vi "DeleteLayer.vi"(6 "error in":errorcluster, 7 "AntsRect":T8, 9 "Data in":T1={"Class"={"Ants"=refnum, "Layer"=refnum, "Templates"=refnum, "Icon"=refnum, "Glyph"=refnum, "Settings"=refnum, "Tools"=refnum, "History"=refnum}, "Ref"={"Add Layer"=refnum, "Remove Layer"=refnum, "Line Text"=[], "Body Text Spec"=refnum, "DNL_Font"=refnum, "glyph path str"=refnum, "templates path str"=refnum, "Arrow Up"=refnum, "Arrow Down"=refnum, "IE VI Ref"=refnum, "Glyphs tree"=refnum, "Templates tree"=refnum, "Layer Icon Text"=refnum, "Layer Template"=refnum, "Body Text"=refnum, "Search Templates"=refnum, "TextMarker"=refnum, "Tab Control"=refnum, "Search Glyphs"=refnum, "Line Color"=refnum, "DNL_Glyphs []"=refnum, "Fill Color"=refnum, "Tools"=refnum, "Icon"=refnum, "Preview"=refnum, "Ants"=refnum, "Terminals"=refnum, "menu reference"=refnum, "LayerNames"=[], "GlyphLoadAnimation"=refnum, "TemplateLoadAnimation"=refnum, "refreshGlyphs"=refnum, "refreshTemplates"=refnum}, "Support"={"AntsRect"={"left"=0, "top"=0, "right"=0, "bottom"=0}, "Mouse Move Coords"={"Horizontal"=0, "Vertical"=0}, "Mouse Down Coords"={"Horizontal"=0, "Vertical"=0}, "Temp Coord"={"Horizontal"=0, "Vertical"=0}, "Action"=enum."Default", "Edge Color"=4914962, "Fill Color"=16860, "Mouse Down?"=FALSE, "Draft Mode?"=FALSE, "Temp Icon"=bytes[3102], "CTRL Pressed"=FALSE, "Move Selection?"=FALSE, "AntsRect Orig"={"left"=0, "top"=0, "right"=0, "bottom"=0}, "Text"="", "TM Set?"=FALSE, "Mouse inside icon?"=FALSE, "Tool (old value)"=0, "Pencil Move Color"=0, "Swap Colors?"=FALSE, "Shift pressed?"=FALSE}}) -> (0 "error out":errorcluster, 3 "Data out":T1={"Class"={"Ants"=refnum, "Layer"=refnum, "Templates"=refnum, "Icon"=refnum, "Glyph"=refnum, "Settings"=refnum, "Tools"=refnum, "History"=refnum}, "Ref"={"Add Layer"=refnum, "Remove Layer"=refnum, "Line Text"=[], "Body Text Spec"=refnum, "DNL_Font"=refnum, "glyph path str"=refnum, "templates path str"=refnum, "Arrow Up"=refnum, "Arrow Down"=refnum, "IE VI Ref"=refnum, "Glyphs tree"=refnum, "Templates tree"=refnum, "Layer Icon Text"=refnum, "Layer Template"=refnum, "Body Text"=refnum, "Search Templates"=refnum, "TextMarker"=refnum, "Tab Control"=refnum, "Search Glyphs"=refnum, "Line Color"=refnum, "DNL_Glyphs []"=refnum, "Fill Color"=refnum, "Tools"=refnum, "Icon"=refnum, "Preview"=refnum, "Ants"=refnum, "Terminals"=refnum, "menu reference"=refnum, "LayerNames"=[], "GlyphLoadAnimation"=refnum, "TemplateLoadAnimation"=refnum, "refreshGlyphs"=refnum, "refreshTemplates"=refnum}, "Support"={"AntsRect"={"left"=0, "top"=0, "right"=0, "bottom"=0}, "Mouse Move Coords"={"Horizontal"=0, "Vertical"=0}, "Mouse Down Coords"={"Horizontal"=0, "Vertical"=0}, "Temp Coord"={"Horizontal"=0, "Vertical"=0}, "Action"=enum."Default", "Edge Color"=4914962, "Fill Color"=16860, "Mouse Down?"=FALSE, "Draft Mode?"=FALSE, "Temp Icon"=bytes[3102], "CTRL Pressed"=FALSE, "Move Selection?"=FALSE, "AntsRect Orig"={"left"=0, "top"=0, "right"=0, "bottom"=0}, "Text"="", "TM Set?"=FALSE, "Mouse inside icon?"=FALSE, "Tool (old value)"=0, "Pencil Move Color"=0, "Swap Colors?"=FALSE, "Shift pressed?"=FALSE}})   [LabVIEW 2020]
uses:
  Class/Ants/Ants.lvclass
  Class/FakedArray/FakedArray.lvclass
  vi.lib/LabVIEW Icon API/lv_icon/Classes/Icon/Icon.lvclass
  Class/Icon Library/Glyph.lvclass
  Class/Settings/Settings.lvclass
  Class/Tools/Tools Paint.lvclass
  History/History/History.lvclass
  vi.lib/LabVIEW Icon API/lv_icon/Classes/Layer/Layer.lvclass
  vi.lib/LabVIEW Icon API/LabVIEW Icon API.lvlib
  lv_icon.lvlib
  History/History.lvlib
  <vilib>/Utility/miscctls.llb/LVPoint32TypeDef.ctl
  Controls/SupportClass_Action.ctl
  vi.lib/LabVIEW Icon API/lv_icon/Controls/IEColor.ctl
  Controls/Support Cluster.ctl
  Controls/References Cluster.ctl
  Controls/IE Classes.ctl
  Controls/Global Data.ctl
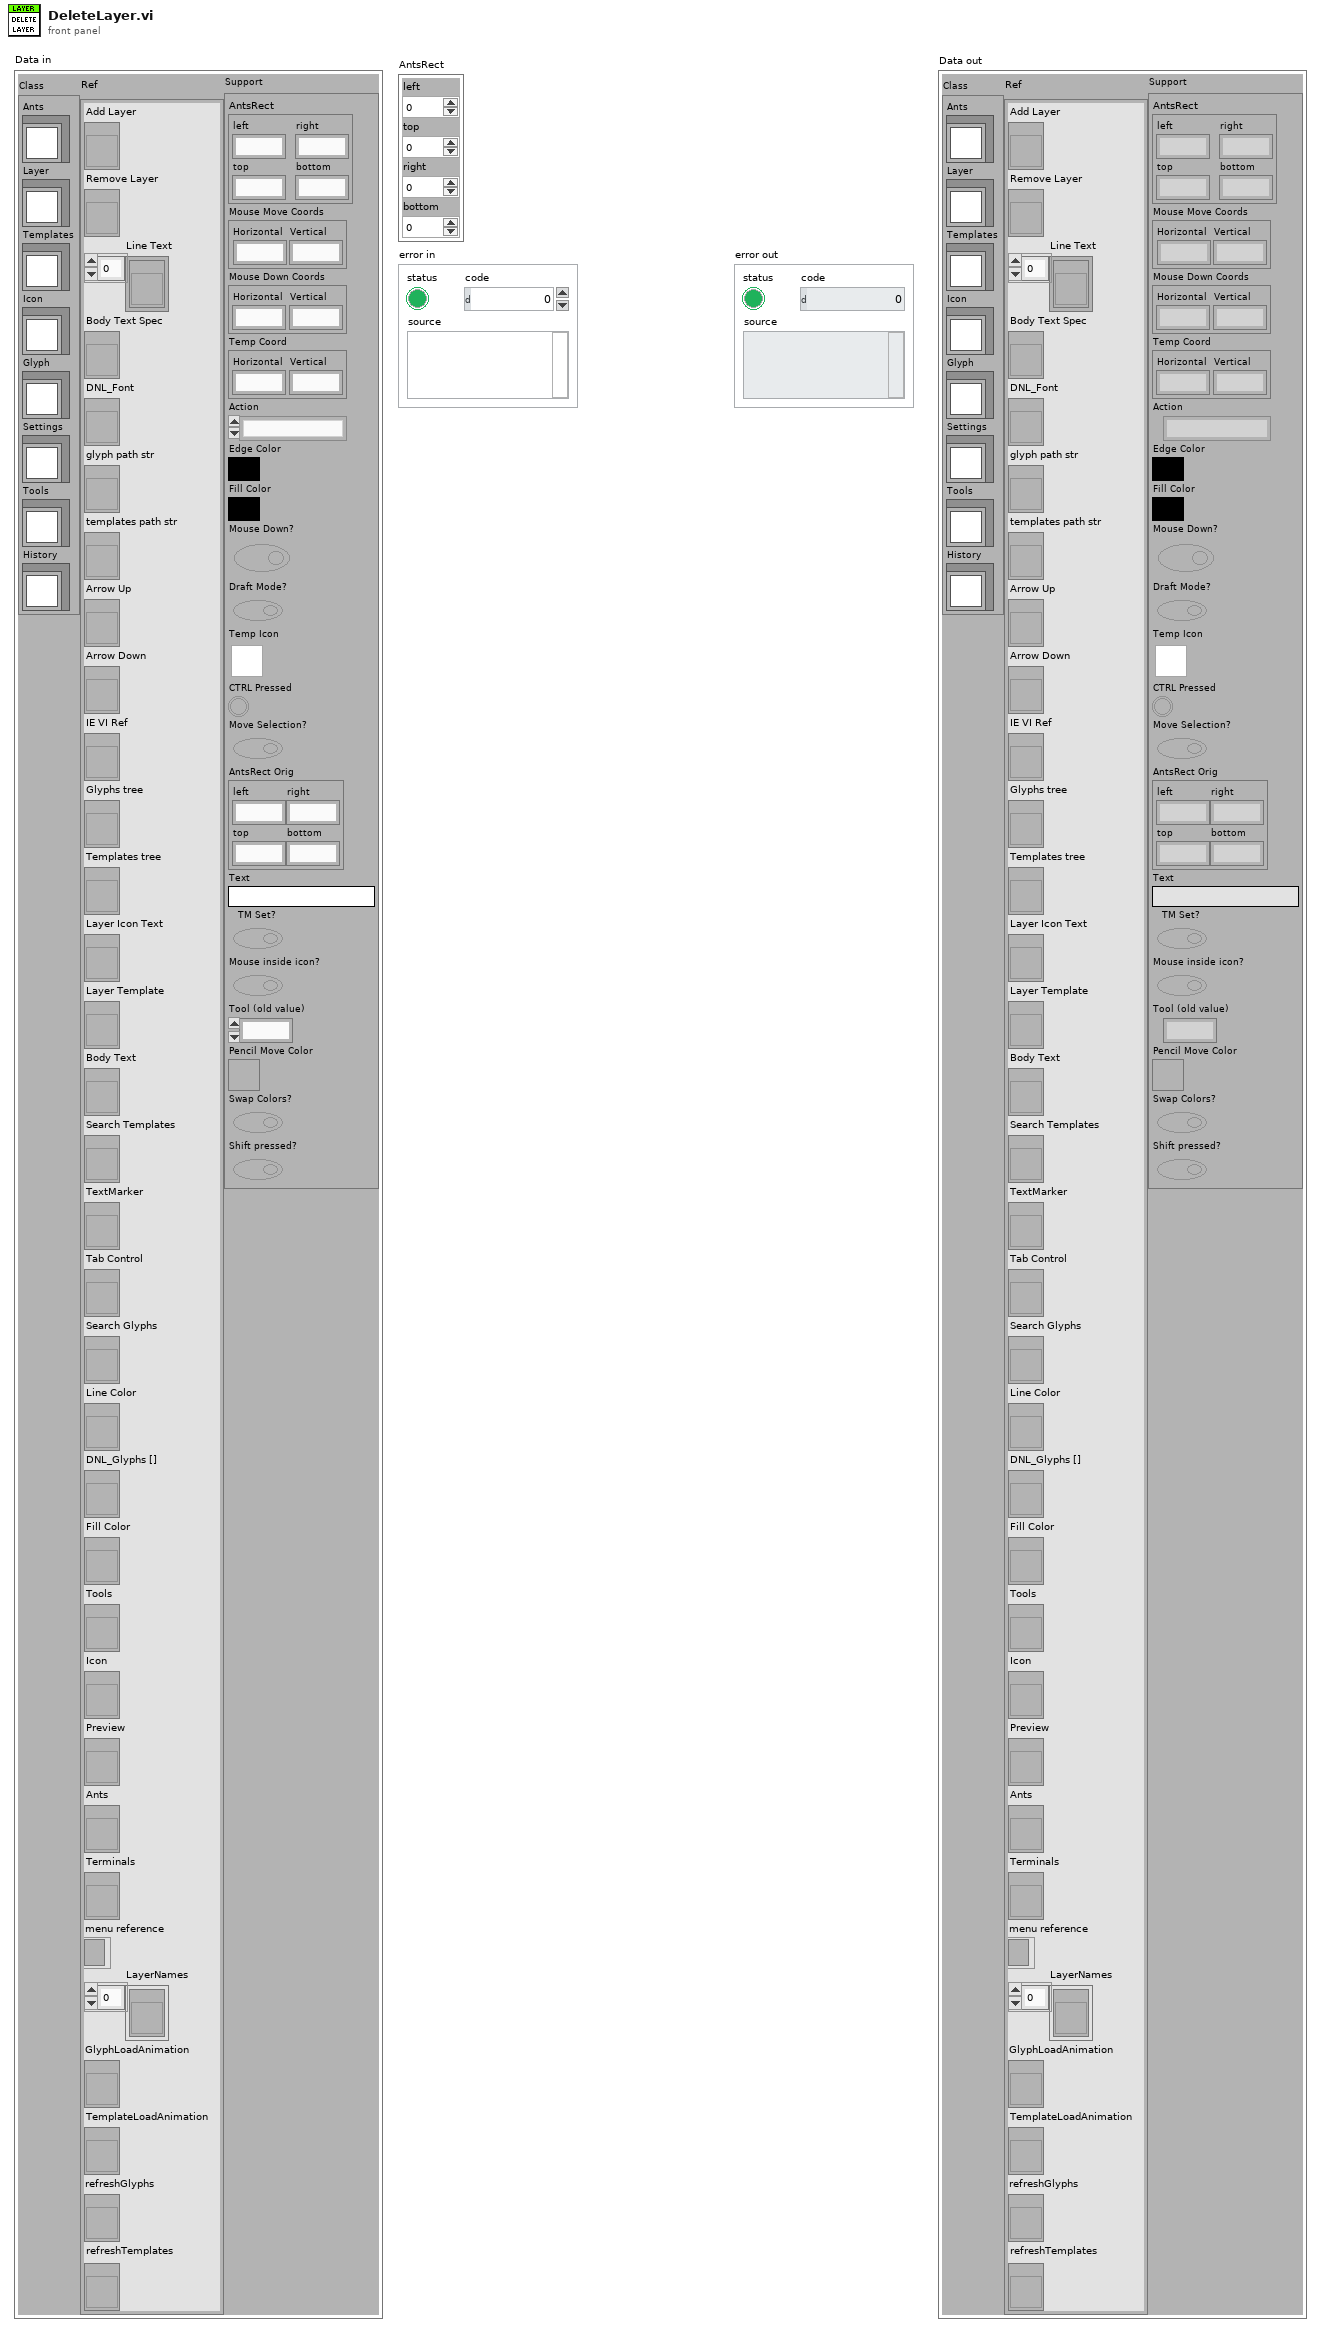
[diagram p1: front panel]
types:
  T1 = typedef "lv_icon.lvlib/Global Data.ctl" = cluster{"Class":T2, "Ref":T3, "Support":T4}
  T2 = typedef "lv_icon.lvlib/IE Classes.ctl" = cluster{"Ants":refnum<class "Ants.lvclass">, "Layer":refnum<class "FakedArray.lvclass">, "Templates":refnum<class "FakedArray.lvclass">, "Icon":refnum<class "Icon.lvclass">, "Glyph":refnum<class "Glyph.lvclass">, "Settings":refnum<class "Settings.lvclass">, "Tools":refnum<class "Tools Paint.lvclass">, "History":refnum<class "History.lvclass">}
  T3 = typedef "lv_icon.lvlib/References Cluster.ctl" = cluster{"Add Layer":refnum<vi>, "Remove Layer":refnum<vi>, "Line Text":refnum<vi>[], "Body Text Spec":refnum<vi>, "DNL_Font":refnum<vi>, "glyph path str":refnum<vi>, "templates path str":refnum<vi>, "Arrow Up":refnum<vi>, "Arrow Down":refnum<vi>, "IE VI Ref":refnum<vi>, "Glyphs tree":refnum<vi>, "Templates tree":refnum<vi>, "Layer Icon Text":refnum<vi>, "Layer Template":refnum<vi>, "Body Text":refnum<vi>, "Search Templates":refnum<vi>, "TextMarker":refnum<vi>, "Tab Control":refnum<vi>, "Search Glyphs":refnum<vi>, "Line Color":refnum<vi>, "DNL_Glyphs []":refnum<vi>, "Fill Color":refnum<vi>, "Tools":refnum<vi>, "Icon":refnum<vi>, "Preview":refnum<vi>, "Ants":refnum<vi>, "Terminals":refnum<vi>, "menu reference":refnum<k9>, "LayerNames":refnum<vi>[], "GlyphLoadAnimation":refnum<vi>, "TemplateLoadAnimation":refnum<vi>, "refreshGlyphs":refnum<vi>, "refreshTemplates":refnum<vi>}
  T4 = typedef "lv_icon.lvlib/Support Cluster.ctl" = cluster{"AntsRect":cluster{"left":i16, "top":i16, "right":i16, "bottom":i16}, "Mouse Move Coords":T5, "Mouse Down Coords":T5, "Temp Coord":T5, "Action":T6, "Edge Color":T7, "Fill Color":T7, "Mouse Down?":bool, "Draft Mode?":bool, "Temp Icon":picture, "CTRL Pressed":bool, "Move Selection?":bool, "AntsRect Orig":cluster{"left":i16, "top":i16, "right":i16, "bottom":i16}, "Text":string, "TM Set?":bool, "Mouse inside icon?":bool, "Tool (old value)":u32, "Pencil Move Color":u32, "Swap Colors?":bool, "Shift pressed?":bool}
  T5 = typedef "LVPoint32TypeDef.ctl" = cluster{"Horizontal":i32, "Vertical":i32}
  T6 = typedef "SupportClass_Action.ctl" = enum16{"Default", "Move Selection", "Glyph Library", "Tool"}
  T7 = typedef "IEColor.ctl" = u32
  T8 = cluster{"left":i16, "top":i16, "right":i16, "bottom":i16}
  T9 = typedef "Layer.ctl" = cluster{"LayerIcon":picture, "LayerName":string, "Opacity":u8, "Visibility?":bool}
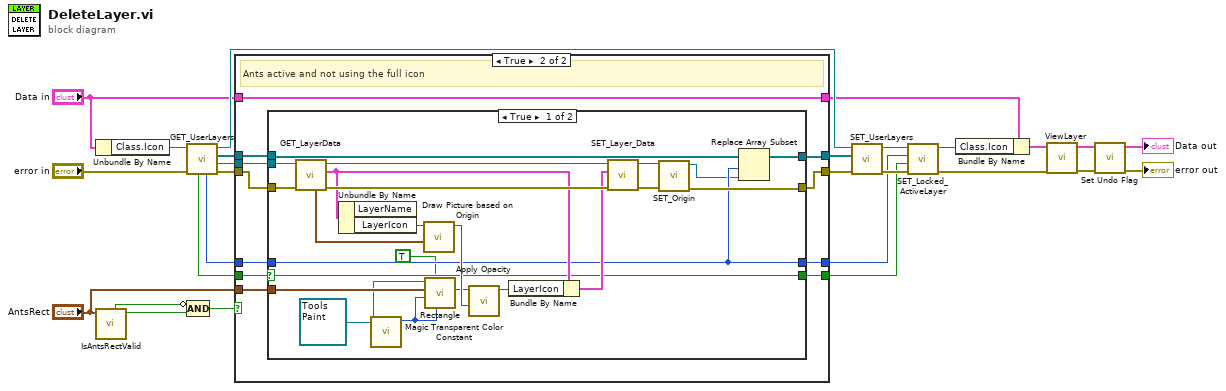
[diagram p0: block diagram]
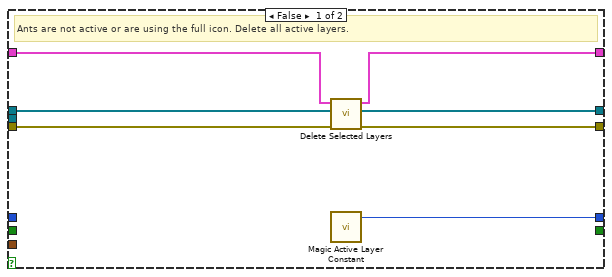
[diagram p2: hidden frame]
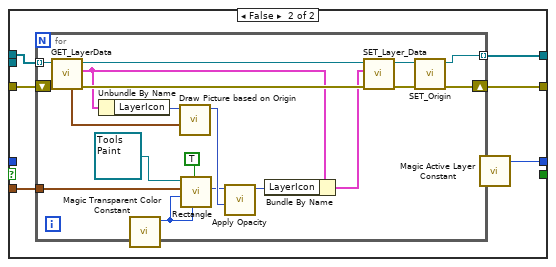
[diagram p3: hidden frame]
diagram:
  n1 = Unbundle By Name("Data in") -> ("Class.Icon"=w12:refnum<class "Icon.lvclass">)
  n2 = call "IsAntsRectValid.vi"("AntsRect"="AntsRect") -> ("Valid?"=w5:bool, "Max. Rect size?"=w4:bool)  [unwired: 9 out]
  n3 = call-dynamic "GET_UserLayers.vi"("error in (no error)"="error in", "Icon.lvclass in"=w12) -> ("error out"=w26:errorcluster, "Active Layer"=w17:refnum<class "Layer.lvclass">, "All Layers"=w18:refnum<class "Layer.lvclass">[], "Icon.lvclass out"=w20:refnum<class "Icon.lvclass">, "#Active Layer"=w19:i32, "Layer Locked?"=w16:bool)  [unwired: 4 out]
  n4 = Compound Arithmetic op=AND(invert w4, w5) -> (w3:bool)
  n5 = case shown="True" w3 {
    tunnel: [w34 w44] -> w27
    tunnel: [w32 w37] -> w6
    tunnel: w19 -> [_ w41]
    tunnel: w26 -> [w33 w45]
    tunnel: w18 -> [w31 w38]
    tunnel: w17 -> [_ w40]
    tunnel: w16 -> [_ w42]
    tunnel: "AntsRect" -> [_ w39]
    tunnel: [w30 w36] -> w14
    tunnel: [_ w35] -> w13
    tunnel: "Data in" -> [w29 w43]
    tunnel: [w28 w43] -> w9
    frame False {
      # "Ants are not active or are using the full icon. Delete all active layers."
      n6 = call "Delete Selected Layers.vi"("error in"=w33, "All Layers in"=w31, "Data in"=w29) -> ("error out"=w34:errorcluster, "All Layers out"=w32:refnum<class "Layer.lvclass">[], "Data out"=w28:T1)  [unwired: 6 in]
      n7 = call "Magic Active Layer Constant.vi"() -> ("Magic Constant"=w30:i32)  [unwired: 19 out]
    }
    frame True {
      # "Ants active and not using the full icon"
      n8 = case shown="True" w42 {
        selector: w42 -> [w51 _]
        tunnel: w41 -> [w52 _]
        tunnel: w40 -> [w64 _]
        tunnel: w45 -> [w68 w74]
        tunnel: w39 -> [w61 w72]
        tunnel: [w66 w73] -> w44
        tunnel: w38 -> [w54 w71]
        tunnel: [w53 w70] -> w37
        tunnel: [w52 w69] -> w36
        tunnel: [w51 _] -> w35
        frame True {
          n9 = call-dynamic "GET_LayerData.vi"("error in (no error)"=w68, "Layer.lvclass in"=w64) -> ("error out"=w65:errorcluster, "Data"=w58:T9, "Layer.lvclass out"=w56:refnum<class "Layer.lvclass">, "Origin"=w62:T5)  [unwired: 6 out]
          n10 = Unbundle By Name(w58) -> ("LayerIcon"=w63:picture)  [unwired: 1 out]
          n11 = call "Magic Transparent Color Constant.vi"() -> ("Magic transparent color constant"=w48:u32)  [unwired: 11 out]
          n12 = call "Draw Picture based on Origin.vi"("Origin"=w62, "LayerIcon in"=w63) -> ("LayerIcon out"=w60:picture)  [unwired: 1 in, 8 out]
          n13 = call-dynamic "Rectangle.vi"("Fill Color"=w48, "fill?(F)"=TRUE, "Edge Color"=w48, "rect"=w61, "Tools Paint in"=refnum<class "Tools Paint.lvclass"> refnum) -> ("new picture"=w59:picture)  [unwired: 1 in, 5 out]
          n14 = call "Apply Opacity.vi"("Bottom"=w60, "Top"=w59) -> ("new picture"=w57:picture)  [unwired: 1 in, 8 out]
          n15 = Bundle By Name(cluster=w58, "LayerIcon"=w57) -> (w55:T9)
          n16 = call-dynamic "SET_Layer_Data.vi"("error in (no error)"=w65, "Data"=w55, "Layer.lvclass in"=w56) -> ("error out"=w67:errorcluster, "Layer.lvclass out"=w47:refnum<class "Layer.lvclass">)  [unwired: 1 in, 6 out]
          n17 = call-dynamic "SET_Origin.vi"("error in"=w67, "Layer.lvclass in"=w47) -> ("error out"=w66:errorcluster, "Layer.lvclass out"=w46:refnum<class "Layer.lvclass">)  [unwired: 8 in]
          n18 = Replace Array Subset(array=w54, new element=w46, index=w52) -> (w53:refnum<class "Layer.lvclass">[])
        }
        frame False {
          n19 = for {
            tunnel: w72 -> [w87]
            shift-right: [w91] -> w73
            shift-left: w74 -> [w93]
            tunnel: w71 -> [w80] mode=indexing
            tunnel: [w75] -> w70 mode=indexing
            n20 = call-dynamic "GET_LayerData.vi"("error in (no error)"=w93, "Layer.lvclass in"=w80) -> ("error out"=w90:errorcluster, "Data"=w84:T9, "Layer.lvclass out"=w82:refnum<class "Layer.lvclass">, "Origin"=w88:T5)  [unwired: 6 out]
            n21 = Unbundle By Name(w84) -> ("LayerIcon"=w89:picture)
            n22 = call "Magic Transparent Color Constant.vi"() -> ("Magic transparent color constant"=w77:u32)  [unwired: 11 out]
            n23 = call "Draw Picture based on Origin.vi"("Origin"=w88, "LayerIcon in"=w89) -> ("LayerIcon out"=w86:picture)  [unwired: 1 in, 8 out]
            n24 = call-dynamic "Rectangle.vi"("Fill Color"=w77, "fill?(F)"=TRUE, "Edge Color"=w77, "rect"=w87, "Tools Paint in"=refnum<class "Tools Paint.lvclass"> refnum) -> ("new picture"=w85:picture)  [unwired: 1 in, 5 out]
            n25 = call "Apply Opacity.vi"("Bottom"=w86, "Top"=w85) -> ("new picture"=w83:picture)  [unwired: 1 in, 8 out]
            n26 = Bundle By Name(cluster=w84, "LayerIcon"=w83) -> (w81:T9)
            n27 = call-dynamic "SET_Layer_Data.vi"("error in (no error)"=w90, "Data"=w81, "Layer.lvclass in"=w82) -> ("error out"=w92:errorcluster, "Layer.lvclass out"=w76:refnum<class "Layer.lvclass">)  [unwired: 1 in, 6 out]
            n28 = call-dynamic "SET_Origin.vi"("error in"=w92, "Layer.lvclass in"=w76) -> ("error out"=w91:errorcluster, "Layer.lvclass out"=w75:refnum<class "Layer.lvclass">)  [unwired: 8 in]
          }
          n29 = call "Magic Active Layer Constant.vi"() -> ("Magic Constant"=w69:i32)  [unwired: 19 out]
        }
      }
    }
  }
  n30 = call-dynamic "SET_UserLayers.vi"("error in"=w27, "Layers"=w6, "Icon.lvclass in"=w20) -> ("error out"=w25:errorcluster, "Icon.lvclass out"=w8:refnum<class "Icon.lvclass">)  [unwired: 7 in]
  n31 = call-dynamic "SET_Locked_ActiveLayer.vi"("error in (no error)"=w25, "Layers Locked?"=w13, "Active Layer"=w14, "Icon.lvclass in"=w8) -> ("error out"=w24:errorcluster, "Icon.lvclass out"=w10:refnum<class "Icon.lvclass">)  [unwired: 6 out]
  n32 = Bundle By Name(cluster=w9, "Class.Icon"=w10) -> (w7:T1)
  n33 = call "ViewLayer.vi"("error in (no error)"=w24, "Data in"=w7) -> ("error out"=w22:errorcluster, "Data out"=w2:T1)  [unwired: 2 in, 6 out]
  n34 = call "Set Undo Flag.vi"("error in"=w22, "Data in"=w2) -> ("error out"=→"error out":errorcluster, "Data out"=→"Data out":T1)  [unwired: 8 in]
